vi "EnhedsOmregner.vi"() -> ()   [LabVIEW 2022 SP3]
uses:
  <vilib>/express/express arith-compare/Formula/XNode/ExpressFormulaBlockNode.xnode
panel:
  out "Output":string
  in  "Input":dbl
  in  "Decimaler":dbl
  in  "Input enhed":bool
  # "°F"
  # "°C"
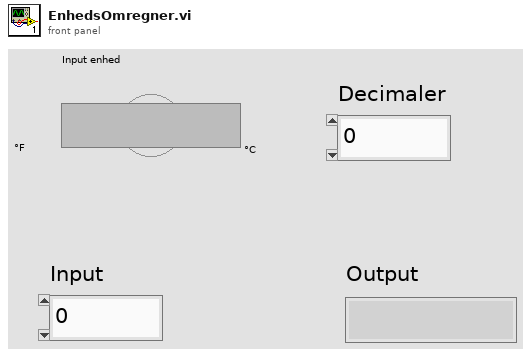
[diagram p1: front panel]
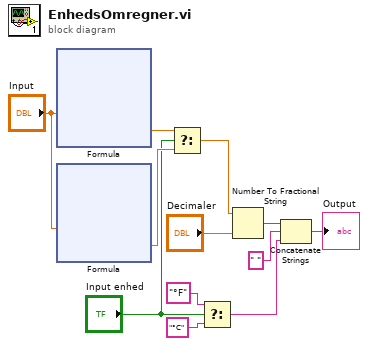
[diagram p0: block diagram]
diagram:
  n1 = xnode "Formula"("T"="Input") -> ("Result"=w12:dbl)  [unwired: 1 in, 1 out]
  n2 = xnode "Formula"("T"="Input") -> ("Result"=w10:dbl)  [unwired: 1 in, 1 out]
  n3 = Select(t=w12, s="Input enhed", f=w10) -> (s? t:f=w8:dbl)
  n4 = Select(t="°F" ("string"), s="Input enhed", f="°C" ("string")) -> (s? t:f=w1:string)
  n5 = Number To Fractional String(number=w8, precision (6)="Decimaler") -> (F-format string=w7:string)  [unwired: 2 in]
  n6 = Concatenate Strings(w7, " " ("string"), w1) -> (→"Output":string)
